vi "WaitNotification.vi"(10 "timeup":i32=-1, 11 "notification":string) -> (3 "massage":string)   [LabVIEW 2011]
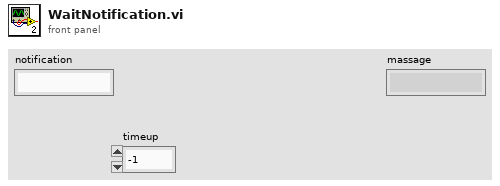
[diagram p1: front panel]
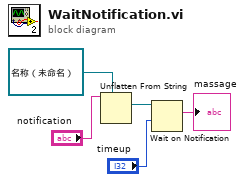
[diagram p0: block diagram]
diagram:
  n1 = Unflatten From String(type=refnum<notifier> refnum ("通知器输出"), binary string="notification") -> (value=w1:refnum<notifier>)  [unwired: 3 in, 2 out]
  n2 = Wait on Notification(notifier=w1, timeout in ms (-1)="timeup") -> (notification=→"massage":string)  [unwired: 2 in, 3 out]
